vi "Flatten to XML (PVI).vi"(8 "error in (no error)":errorcluster, 10 "indent levels":i32, 11 "Variant":variant) -> (0 "error out":errorcluster, 3 "XML":string)   [LabVIEW 2018, in "XML Config.lvlib"]
doc: "This VI is used to facilitate saving XML files of arbitrary simple clusters (i.e one\nthat does not contain arrays of clusters) as config files and then reading them\nback even though the cluster may have been updated (may added or removed\ncontrols from the cluster)."
uses:
  XML Config.lvlib
  <userlib>/_OpenG.lib/lvdata/lvdata.llb/Type Descriptor Enumeration__ogtk.ctl
  Utilities/ISO 8601 type.ctl
  <vilib>/Waveform/WDTOps.llb/WDT Waveform to XY Pairs DBL.vi
panel:
  out "Enum Strings":string[](array[string])
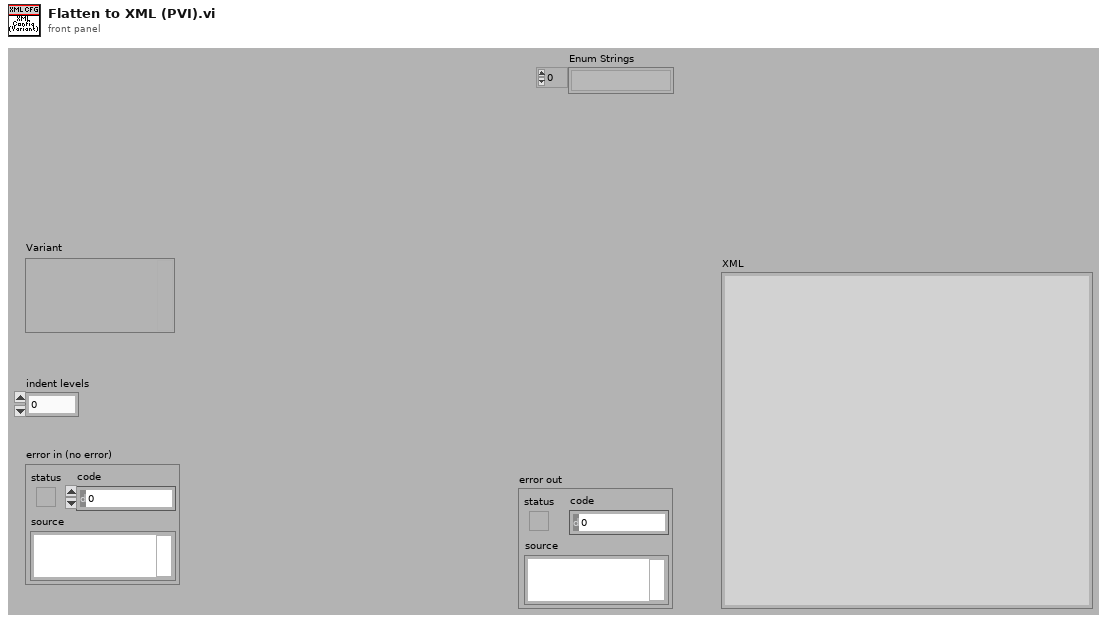
[diagram p1: front panel]
types:
  T1 = typedef "Type Descriptor Enumeration__ogtk.ctl" = enum8{"<Null>", "I8", "I16", "I32", "I64", "U8", "U16", "U32", "U64", "SGL", "DBL", "EXT", "CSG", "CDB", "CXT", "0x0F", "0x10", "0x11", "0x12", "0x13", "0x14", "Enum U8", "Enum U16", "Enum U32", "Enum U64", "SGL PQ", "DBL PQ", "EXT PQ", "CSG PQ", "CDB PQ", "CXT PQ", "0x1F", "0x20", "Boolean", "0x22", "0x23", "0x24", "0x25", "0x26", "0x27", "0x28", "0x29", "0x2A", "0x2B", "0x2C", "0x2D", "0x2E", "0x2F", "String", "0x31", "Path", "Pict", "0x34", "0x35", "0x36", "DAQ", "0x38", "0x39", "0x3A", "0x3B", "0x3C", "0x3D", "0x3E", "0x3F", "Array", "0x41", "0x42", "0x43", "0x44", "0x45", "0x46", "0x47", "0x48", "0x49", "0x4A", "0x4B", "0x4C", "0x4D", "0x4E", "0x4F", "Cluster", "0x51", "0x52", "Variant", "Waveform", "0x55", "0x56", "0x57", "0x58", "0x59", "0x5A", "0x5B", "0x5C", "0x5D", "0x5E", "0x5F", "0x60", "0x61", "0x62", "0x63", "0x64", "0x65", "0x66", "0x67", "0x68", "0x69", "0x6A", "0x6B", "0x6C", "0x6D", "0x6E", "0x6F", "Refnum"}
  T2 = typedef "ISO 8601 type.ctl" = enum16{"full ISO 8601 UTC", "basic ISO8601 local", "Windows ISO 8601 UTC", "YYYY-MM-DD UTC", "full ISO 8601 local"}
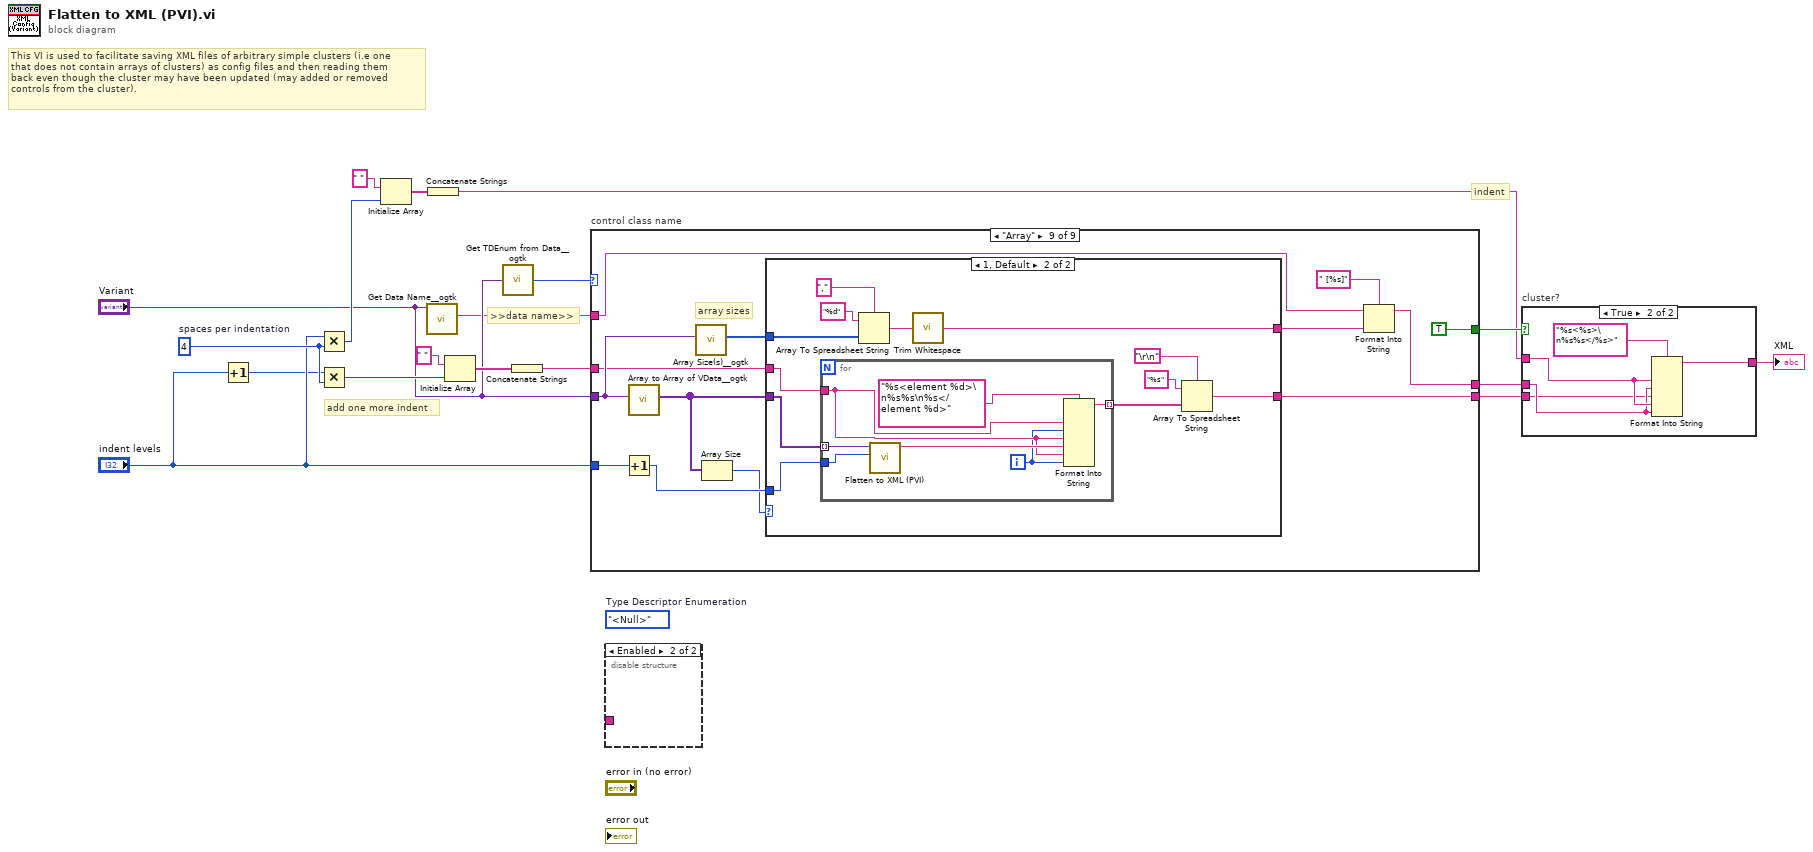
[diagram p0: block diagram]
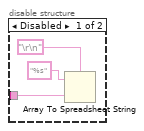
[diagram p2: hidden frame]
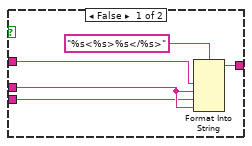
[diagram p3: hidden frame]
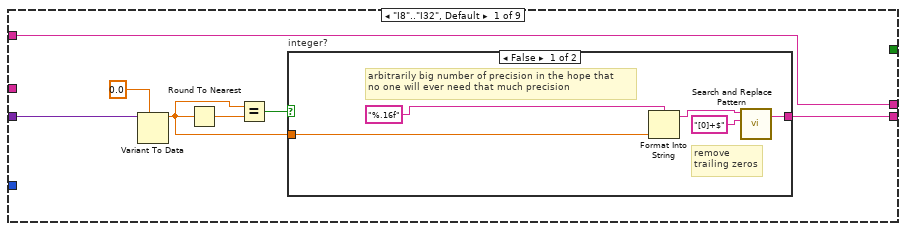
[diagram p4: hidden frame]
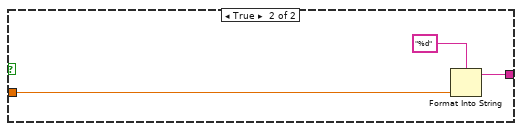
[diagram p5: hidden frame]
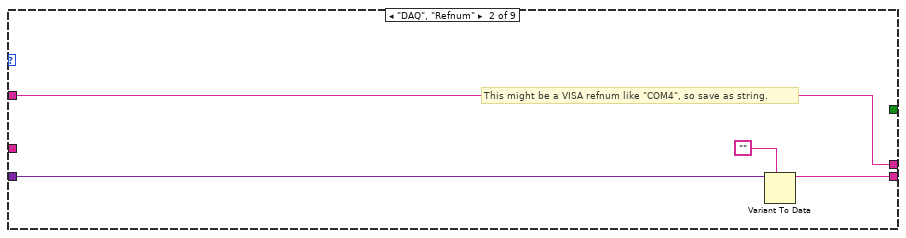
[diagram p6: hidden frame]
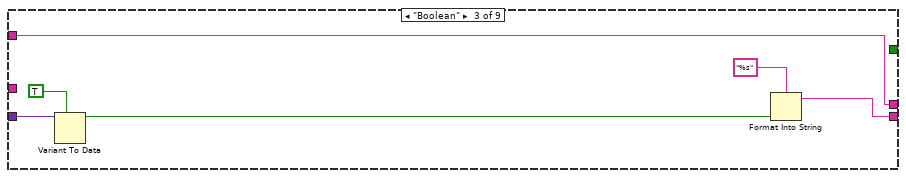
[diagram p7: hidden frame]
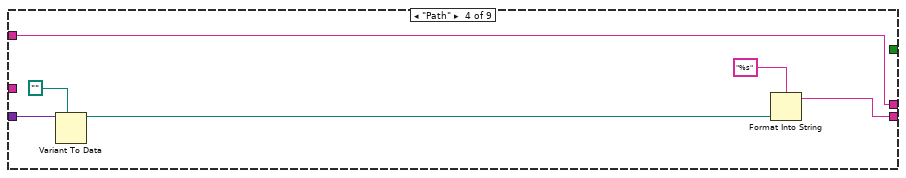
[diagram p8: hidden frame]
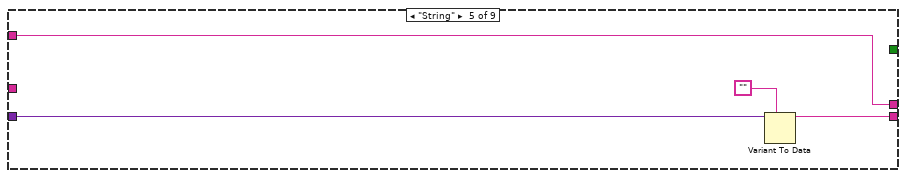
[diagram p9: hidden frame]
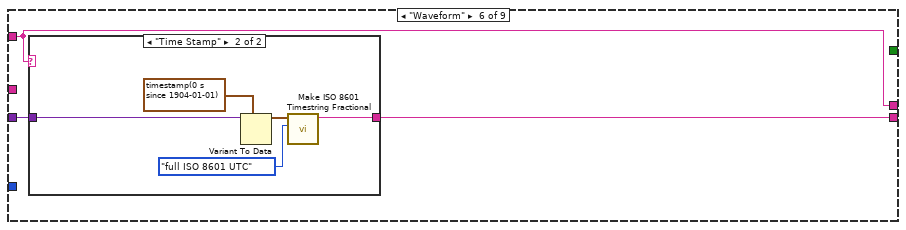
[diagram p10: hidden frame]
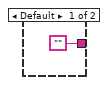
[diagram p11: hidden frame]
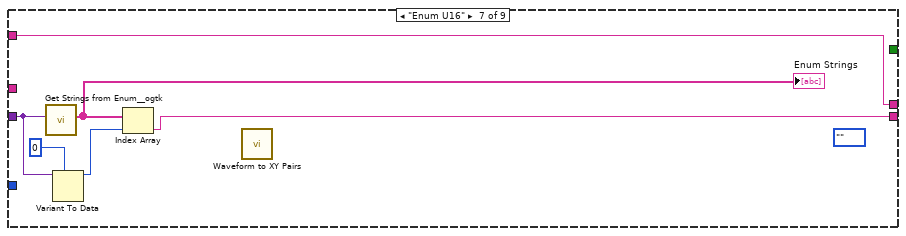
[diagram p12: hidden frame]
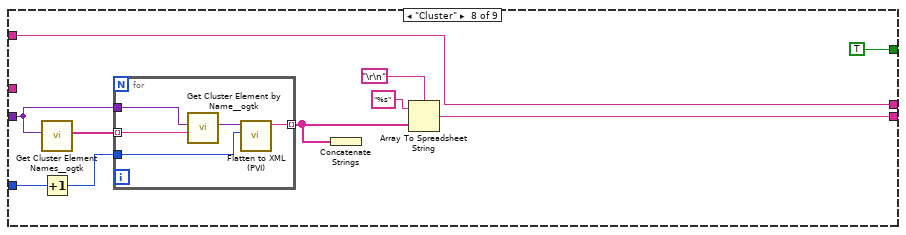
[diagram p13: hidden frame]
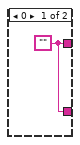
[diagram p14: hidden frame]
diagram:
  (unwired) Type_Descriptor_Enumeration__ogtk."<Null>"  # Type Descriptor Enumeration
  w7 = 4  # spaces per indentation
  # "This VI is used to facilitate saving XML files of arbitrary simple clusters (i.e one\nthat does not contain arrays of clusters) as config files and then reading them\nback even though the cluster may have been updated (may added or removed\ncontrols from the cluster)."
  # ">>data name>>"
  # "add one more indent"
  # "indent"
  n1 = Increment(x="indent levels") -> (x+1=w5:i32)
  n2 = Multiply(x="indent levels", y=w7) -> (x*y=w16:i32)
  n3 = Multiply(x=w5, y=w7) -> (x*y=w10:i32)
  n4 = Initialize Array(" " ("format string"), w16) -> (w17:string[])
  n5 = call <userlib>:"Get Data Name__ogtk.vi"("Data"="Variant") -> ("Data Name"=w2:string)  [unwired: 8 in, 2 out]
  n6 = Concatenate Strings(w17) -> (w11:string)
  n7 = Initialize Array(" " ("format string"), w10) -> (w9:string[])
  n8 = call <userlib>:"Get TDEnum from Data__ogtk.vi"("Data"="Variant") -> ("Type Descriptor Enumeration"=w15:T1)  [unwired: 4 in]
  n9 = Concatenate Strings(w9) -> (w4:string)
  n10 = case "control class name" shown="\"Array\"" w15 {
    tunnel: "Variant" -> [w25 w37 w43 w49 w53 w56 w68 w74 w90]
    tunnel: [w20 w34 w39 w45 w51 w55 w64 w70 w91] -> w14
    tunnel: "indent levels" -> [_ _ _ _ _ _ _ w78 w96]
    tunnel: [_ _ _ _ _ _ _ TRUE TRUE] -> w13
    tunnel: w4 -> [_ _ _ _ _ _ _ _ w89]
    tunnel: [w19 w36 w38 w44 w50 w54 w67 w69 w86] -> w1
    tunnel: w2 -> [w19 w36 w38 w44 w50 w54 w67 w69 w87]
    frame "I8".."I32", Default {
      n11 = Variant To Data(type=0.0, Variant=w25) -> (data=w23:dbl)  [unwired: 1 in, 1 out]
      n12 = Round To Nearest(number=w23) -> (nearest integer value=w22:dbl)
      n13 = Equal?(x=w23, y=w22) -> (x = y?=w21:bool)
      n14 = case "integer?" shown="False" w21 {
        tunnel: [w26 w31] -> w20
        tunnel: w23 -> [w29 w33]
        frame False {
          # "arbitrarily big number of precision in the hope that\nno one will ever need that much precision"
          # "remove\ntrailing zeros"
          n15 = Format Into String(format string="%.16f", w29) -> (resulting string=w27:string)  [unwired: 2 in, 1 out]
          n16 = call <vilib>:"Search and Replace Pattern.vi"("string"=w27, "regular expression (\"\")"="[0]+$" ("regular expression (\"\")")) -> ("result string"=w26:string)  [unwired: 3 in, 1 out]
        }
        frame True {
          n17 = Format Into String(format string="%d", w33) -> (resulting string=w31:string)  [unwired: 2 in, 1 out]
        }
      }
    }
    frame "DAQ", "Refnum" {
      # "This might be a VISA refnum like \"COM4\", so save as string."
      n18 = Variant To Data(type="", Variant=w37) -> (data=w34:string)  [unwired: 1 in, 1 out]
    }
    frame "Boolean" {
      n19 = Variant To Data(type=TRUE, Variant=w43) -> (data=w41:bool)  [unwired: 1 in, 1 out]
      n20 = Format Into String(format string="%s", w41) -> (resulting string=w39:string)  [unwired: 2 in, 1 out]
    }
    frame "Path" {
      n21 = Variant To Data(type=path "", Variant=w49) -> (data=w46:path)  [unwired: 1 in, 1 out]
      n22 = Format Into String(format string="%s", w46) -> (resulting string=w45:string)  [unwired: 2 in, 1 out]
    }
    frame "String" {
      n23 = Variant To Data(type="", Variant=w53) -> (data=w51:string)  [unwired: 1 in, 1 out]
    }
    frame "Waveform" {
      n24 = case shown="\"Time Stamp\"" w54 {
        tunnel: w56 -> [_ w59]
        tunnel: ["" w58] -> w55
        frame Default {
        }
        frame "Time Stamp" {
          n25 = Variant To Data(type=timestamp(0 s since 1904-01-01), Variant=w59) -> (data=w60:timestamp)  [unwired: 1 in, 1 out]
          n26 = call "Make ISO 8601 Timestring Fractional.vi"("ISO 8601 type"=ISO_8601_type."full ISO 8601 UTC", "Time Stamp"=w60) -> ("ISO 8601 Timestring"=w58:string)  [unwired: 8 in, 1 out]
        }
      }
    }
    frame "Enum U16" {
      (unwired) enum16{""}.""
      n27 = call <userlib>:"Get Strings from Enum__ogtk.vi"("Enum"=w68) -> ("Enum Strings"=w66:string[])  [unwired: 7 in, 3 out]
      "Enum Strings" <- w66
      n28 = Variant To Data(type=u16 0 ("unsigned 16bit integer"), Variant=w68) -> (data=w65:u16)  [unwired: 1 in, 1 out]
      n29 = Index Array(array=w66, index=w65) -> (element=w64:string)
      n30 = call-poly <vilib>:"Waveform to XY Pairs.vi"() -> ()  [unwired: 9 in, 3 out]
    }
    frame "Cluster" {
      n31 = call <userlib>:"Get Cluster Element Names__ogtk.vi"("Cluster"=w74) -> ("Element Names"=w75:string[])  [unwired: 9 in, 1 out]
      n32 = Increment(x=w78) -> (x+1=w77:i32)
      n33 = for {
        tunnel: w77 -> [w83]
        tunnel: [w82] -> w71 mode=indexing
        tunnel: w75 -> [w81] mode=indexing
        tunnel: w74 -> [w80]
        n34 = call <userlib>:"Get Cluster Element by Name__ogtk.vi"("Element Name"=w81, "Cluster"=w80) -> ("VElement"=w79:variant)  [unwired: 7 in, 2 out]
        n35 = call "Flatten to XML (PVI).vi"("indent levels"=w83, "Variant"=w79) -> ("XML"=w82:string)  [unwired: 8 in, 1 out]
      }
      n36 = Concatenate Strings(w71) -> ()  [unwired: 1 out]
      n37 = Array To Spreadsheet String(delimiter (Tab)="\r\n", array=w71, 3:"%s" ("format string")) -> (spreadsheet string=w70:string)
    }
    frame "Array" {
      # "array sizes"
      n38 = Increment(x=w96) -> (x+1=w94:i32)
      n39 = call <userlib>:"Array to Array of VData__ogtk.vi"("MultiD Array"=w90) -> ("1D Array of Variants"=w92:variant[])  [unwired: 9 in, 1 out]
      n40 = call <userlib>:"Array Size(s)__ogtk.vi"("Array"=w90) -> ("Size(s)"=w88:u32[])  [unwired: 8 in, 2 out]
      n41 = Array Size(array=w92) -> (size(s)=w93:i32)
      n42 = case shown="1, Default" w93 {
        tunnel: [w97 w104] -> w91
        tunnel: w94 -> [_ w109]
        tunnel: w92 -> [_ w108]
        tunnel: w89 -> [_ w103]
        tunnel: w88 -> [_ w102]
        tunnel: [w97 w98] -> w84
        frame 0 {
          w97 = ""
        }
        frame 1, Default {
          n43 = for {
            tunnel: [w113] -> w105 mode=indexing
            tunnel: w109 -> [w116]
            tunnel: w108 -> [w115] mode=indexing
            tunnel: w103 -> [w111]
            i -> [w110]
            n44 = call "Flatten to XML (PVI).vi"("indent levels"=w116, "Variant"=w115) -> ("XML"=w112:string)  [unwired: 8 in, 1 out]
            n45 = Format Into String(format string="%s<element %d>\n%s%s\n%s</element %d>", w111, w110, w111, w112, w111, w110) -> (resulting string=w113:string)  [unwired: 2 in, 1 out]
          }
          n46 = Array To Spreadsheet String(delimiter (Tab)=",", array=w102, 3:"%d" ("format string")) -> (spreadsheet string=w99:string)
          n47 = call <vilib>:"Trim Whitespace.vi"("string"=w99) -> ("trimmed string"=w98:string)  [unwired: 1 in]
          n48 = Array To Spreadsheet String(delimiter (Tab)="\r\n", array=w105, 3:"%s" ("format string")) -> (spreadsheet string=w104:string)
        }
      }
      n49 = Format Into String(format string=" [%s]", initial string=w87, w84) -> (resulting string=w86:string)  [unwired: 1 in, 1 out]
    }
  }
  n50 = disable-structure shown="Enabled" {
    disable-tunnel: _ -> [w117 _]
    frame Disabled {
      n51 = Array To Spreadsheet String(delimiter (Tab)="\r\n", array=w117, 3:"%s" ("format string")) -> ()  [unwired: 1 out]
    }
    frame Enabled {
    }
  }
  n52 = case "cluster?" shown="True" w13 {
    tunnel: [w123 w128] -> w12
    tunnel: w14 -> [w120 w125]
    tunnel: w1 -> [w122 w126]
    tunnel: w11 -> [w121 w127]
    frame False {
      n53 = Format Into String(format string="%s<%s>%s</%s>", w121, w122, w120, w122) -> (resulting string=w123:string)  [unwired: 2 in, 1 out]
    }
    frame True {
      n54 = Format Into String(format string="%s<%s>\n%s%s</%s>", w127, w126, w125, w127, w126) -> (resulting string=w128:string)  [unwired: 2 in, 1 out]
    }
  }
  "XML" <- w12
